vi "set parameters.vi"(10 "parameters":variant, 11 "action in":refnum<class "action.lvclass">) -> (3 "action out":refnum<class "action.lvclass">)   [LabVIEW 2013, in "action.lvclass"]
uses:
  action.lvclass
  action.lvclass/action.ctl
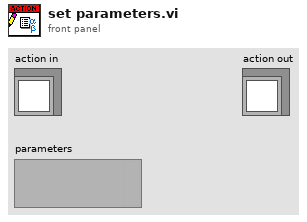
[diagram p1: front panel]
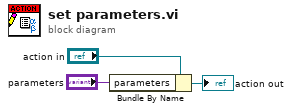
[diagram p0: block diagram]
diagram:
  n1 = Bundle By Name(cluster="action in", "parameters"="parameters") -> (→"action out":refnum<class "action.lvclass">)
